vi "Timing Message Loop.vi"(8 "error in (no error)":errorcluster, 10 "Timers":T1, 11 "Message Queues":T2) -> (0 "error out":errorcluster)   [LabVIEW 2017, in "Message Queue.lvlib"]
uses:
  Message Queue.lvlib
  All Message Queues.ctl
  Message Cluster.ctl
  Acquisition/Acquisition State.ctl
  11995cb8-e311-3fce-f8c0-29dfdff9c03f.vi
  controls/ExitGlobal.vi
  Enqueue Message (Single).vi
  <vilib>/Utility/error.llb/Error Cluster From Error Code.vi
  <vilib>/ErrorRing/Error Ring.xnode
  Acquisition/Acquisition.lvlib
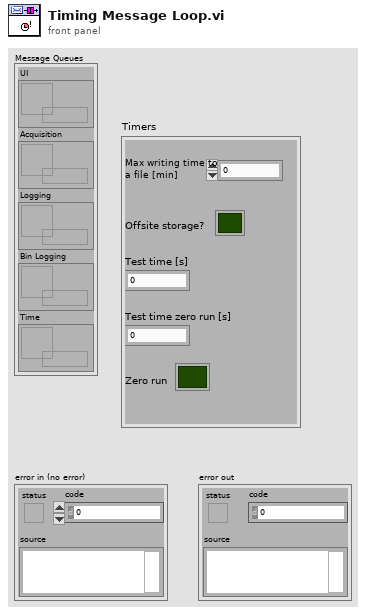
[diagram p1: front panel]
types:
  T1 = cluster{"Offsite storage?":bool, "Test time [s]":dbl, "Test time zero run [s] ":dbl, "Max writing time to a file [min]":dbl, "Zero run":bool}
  T2 = typedef "Message Queue.lvlib/All Message Queues.ctl" = cluster{"UI":refnum<queue>, "Acquisition":refnum<queue>, "Logging":refnum<queue>, "Bin Logging":refnum<queue>, "Time":refnum<queue>}
  T3 = typedef "Acquisition.lvlib/Acquisition State.ctl" = enum16{"Idle", "Acquiring"}
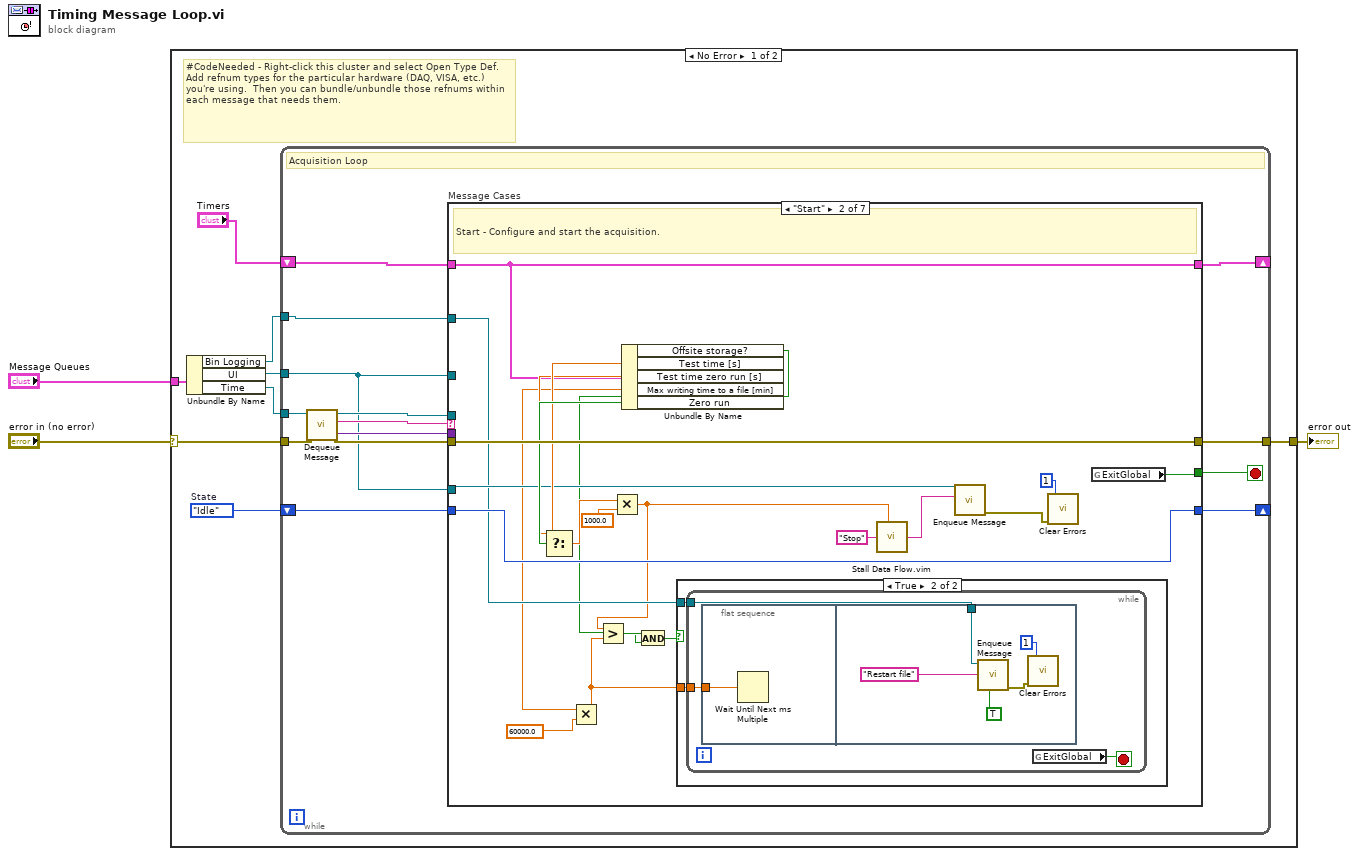
[diagram p0: block diagram]
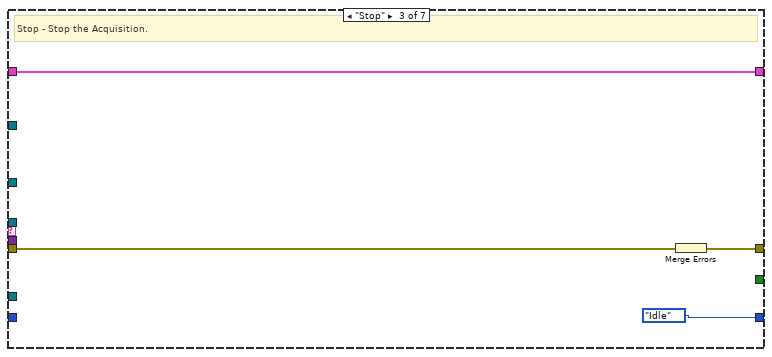
[diagram p4: hidden frame]
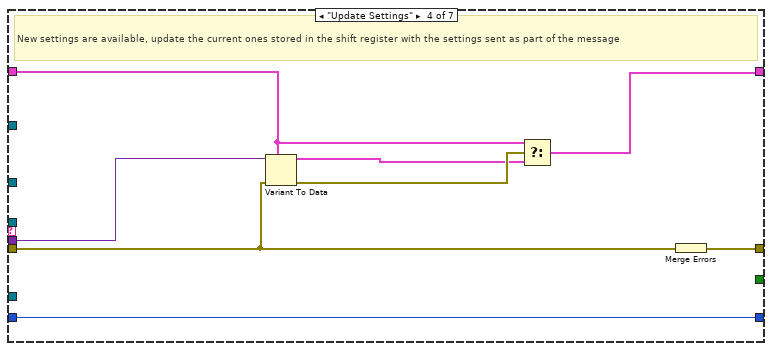
[diagram p5: hidden frame]
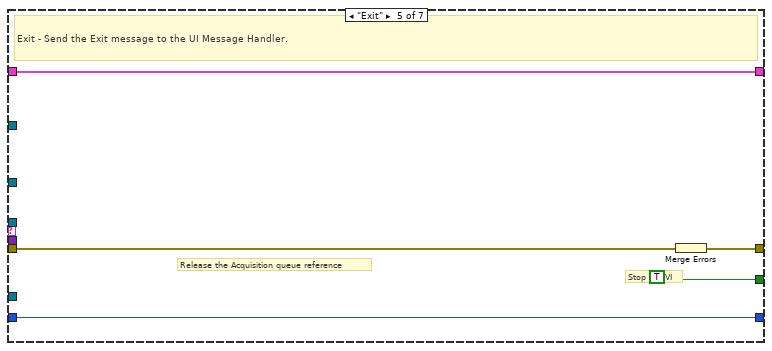
[diagram p6: hidden frame]
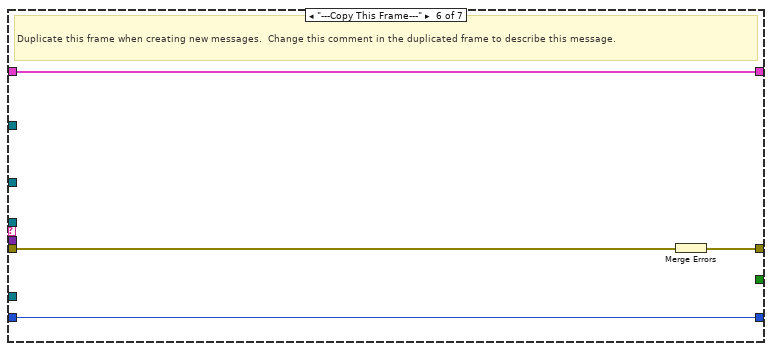
[diagram p7: hidden frame]
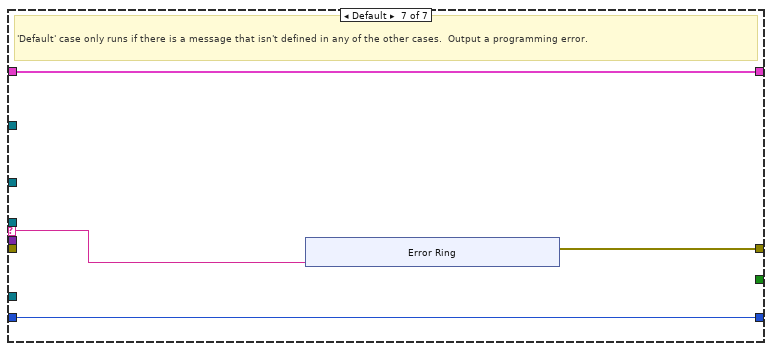
[diagram p8: hidden frame]
diagram:
  n1 = case shown="No Error" "error in (no error)" {
    selector: "error in (no error)" -> [w9 w94]
    tunnel: "Message Queues" -> [w11 _]
    tunnel: [w5 w94] -> w2
    frame No Error {
      w7 = Acquisition_State."Idle"  # State
      # "#CodeNeeded - Right-click this cluster and select Open Type Def.  Add refnum types for the particular hardware (DAQ, VISA, etc.) you're using.  Then you can bundle/unbundle those refnums within each message that needs them."
      n2 = Unbundle By Name(w11) -> ("Bin Logging"=w4:refnum<queue>, "UI"=w8:refnum<queue>, "Time"=w10:refnum<queue>)
      n3 = while {
        tunnel: w10 -> [w18]
        shift-right: [w24] -> _
        shift-left: "Timers" -> [w25]
        tunnel: w8 -> [w14]
        shift-right: [w16] -> _
        shift-left: w7 -> [w17]
        tunnel: w9 -> [w22]
        tunnel: [w13] -> w5
        tunnel: w4 -> [w12]
        stop <- w23 stop-if-true
        # "Acquisition Loop"
        n4 = call "Dequeue Message.vi"("error in (no error)"=w22, "Message Queue"=w18) -> ("error out"=w21:errorcluster, "Message Data"=w19:variant, "Message"=w20:string, "dup Message Queue"=w15:refnum<queue>)  [unwired: 6 in]
        n5 = case "Message Cases" shown="\"Start\"" w20 {
          selector: w20 -> [_ _ _ _ _ _ w83]
          tunnel: w15 -> [_ _ _ _ _ _ _]
          tunnel: w21 -> [w28 w50 w63 w69 w74 w82 _]
          tunnel: [w28 w50 w65 w73 w77 w80 w84] -> w13
          tunnel: w25 -> [w27 w45 w64 w66 w76 w81 w86]
          tunnel: [w27 w45 w64 w70 w76 w81 w86] -> w24
          tunnel: [_ w37 _ _ TRUE _ _] -> w23
          tunnel: w19 -> [_ _ _ w67 _ _ _]
          tunnel: w14 -> [_ _ _ _ _ _ _]
          tunnel: w17 -> [w26 w49 _ w68 w75 w79 w85]
          tunnel: [w26 w49 Acquisition_State."Idle" ("State") w68 w75 w79 w85] -> w16
          tunnel: w14 -> [_ w40 _ _ _ _ _]
          tunnel: w12 -> [_ w36 _ _ _ _ _]
          frame "Initialize" {
            # "Initialize  - Initialize is currently a no-op.  The hardware initialization takes place in the 'Start' message."
          }
          frame "Start" {
            # "Start - Configure and start the acquisition."
            n6 = Unbundle By Name(w45) -> ("Offsite storage?"=w29:bool, "Test time [s]"=w47:dbl, "Test time zero run [s]"=w46:dbl, "Max writing time to a file [min]"=w35:dbl, "Zero run"=w48:bool)
            n7 = Select(t=w46, s=w48, f=w47) -> (s? t:f=w43:dbl)
            n8 = Multiply(x=w35, y=60000.0) -> (x*y=w30:dbl)
            n9 = Multiply(x=w43, y=1000.0) -> (x*y=w31:dbl)
            n10 = Greater?(x=w31, y=w30) -> (0:w32:bool)
            n11 = And(x=w32, y=w29) -> (x .and. y?=w33:bool)
            n12 = case shown="True" w33 {
              tunnel: w36 -> [_ w52]
              tunnel: w30 -> [_ w51]
              frame False {
              }
              frame True {
                n13 = while {
                  tunnel: w52 -> [w55]
                  tunnel: w51 -> [w54]
                  stop <- w53 stop-if-true
                  n14 = flat-sequence {
                    tunnel: w54 -> [w56]
                    tunnel: w55 -> [w58]
                    frame #0 {
                      n15 = Wait Until Next ms Multiple(millisecond multiple=w56) -> ()  [unwired: 1 out]
                    }
                    frame #1 {
                      n16 = call-poly "Enqueue Message.vi"("Priority Message? (F)"=TRUE, "Message"="Restart file" ("t"), "Message Queue"=w58) -> ("error out"=w61:errorcluster)  [unwired: 7 in, 1 out]
                      n17 = call <vilib>:"Clear Errors.vi"("error in (no error)"=w61, "specific error code to clear (0: all)"=1) -> ()  [unwired: 4 in, 2 out]
                    }
                  }
                  n18 = global read "ExitGlobal.vi" "ExitGlobal"() -> (w53:bool)
                }
              }
            }
            n19 = call "Stall Data Flow.vim"("value in"="Stop", "milliseconds to wait"=w31) -> ("value out"=w42:string)  [unwired: 1 out]
            n20 = call-poly "Enqueue Message.vi"("Message"=w42, "Message Queue"=w40) -> ("error out"=w38:errorcluster)  [unwired: 8 in, 1 out]
            n21 = call <vilib>:"Clear Errors.vi"("error in (no error)"=w38, "specific error code to clear (0: all)"=1) -> ()  [unwired: 4 in, 2 out]
            n22 = global read "ExitGlobal.vi" "ExitGlobal"() -> (w37:bool)
          }
          frame "Stop" {
            # "Stop - Stop the Acquisition."
            n23 = Merge Errors(w63) -> (w65:errorcluster)
          }
          frame "Update Settings" {
            # "New settings are available, update the current ones stored in the shift register with the settings sent as part of the message"
            n24 = Variant To Data(error in=w69, type=w66, Variant=w67) -> (data=w71:T1, error out=w72:errorcluster)
            n25 = Select(t=w66, s=w72, f=w71) -> (s? t:f=w70:T1)
            n26 = Merge Errors(w69) -> (w73:errorcluster)
          }
          frame "Exit" {
            # "Release the Acquisition queue reference"
            # "Stop the VI"
            # "Exit - Send the Exit message to the UI Message Handler."
            n27 = Merge Errors(w74) -> (w77:errorcluster)
          }
          frame "---Copy This Frame---" {
            # "Duplicate this frame when creating new messages.  Change this comment in the duplicated frame to describe this message."
            n28 = Merge Errors(w82) -> (w80:errorcluster)
          }
          frame Default {
            # "'Default' case only runs if there is a message that isn't defined in any of the other cases.  Output a programming error."
            n29 = xnode "Error Ring"("parameter 0"=w83) -> ("error out"=w84:errorcluster)
          }
        }
      }
    }
    frame Error {
    }
  }
  "error out" <- w2
